vi "Pressure_statistic with temperature.vi"() -> ()   [LabVIEW 2014]
uses:
  <vilib>/Utility/error.llb/DialogType.ctl
  <instrlib>/Fluke 884X Series/Public/Data/Read (Single Point).vi
  Instance          11 26Saved   Pressure_statistic .vi
  Instance           1 26Saved   Pressure_statistic .vi
  Instance           7 26Saved   Pressure_statistic .vi
  Instance           6 26Saved   Pressure_statistic .vi
  Instance          18 26Saved   Pressure_statistic .vi
  Instance           2 26Saved   Pressure_statistic .vi
  Instance           5 26Saved   Pressure_statistic .vi
  <vilib>/Utility/file.llb/Write To Spreadsheet File (DBL).vi
  Instance           4 26Saved   Pressure_statistic .vi
  Instance           9 26Saved   Pressure_statistic .vi
  Instance           8 26Saved   Pressure_statistic .vi
  Instance          17 26Saved   Pressure_statistic .vi
  Instance          16 26Saved   Pressure_statistic .vi
  <instrlib>/Fluke 884X Series/Fluke 884X Series.lvlib
panel:
  out "Temperature from Fluke884X":dbl(graph)
  out "Temperature,V":dbl
  in  "VISA resource name":refnum<visa-resource-name>
  in  "Wire Mode (1: 4-Wire)":i16(ring)=1 items=["2-Wire", "4-Wire"]
  in  "Unit (0: Celsius)":u16(ring) items=["C", "F", "K"]
  in  "RTD Type (0: PT100_385)":u16(ring) items=["PT100_385", "PT100_392", "Custom"]
  in  "R0 (100 ohms)":i32=100
  in  "Serial Configuration":T1={"Baud Rate"=9600, "Parity"=0, "Data Bits"=8, "Stop Bits"=10, "Flow Control"=0} {"Flow Control" items=["None", "XON/XOFF", "RTS/CTS", "XON/XOFF & RTS/CTS", "DTR/DSR", "XON/XOFF & DTR/DSR"]; "Stop Bits" items=["1.0"=10, "1.5"=15, "2.0"=20]; "Data Bits" items=["7"=7, "8"=8]; "Parity" items=["None", "Odd", "Even", "Mark", "Space"]; "Baud Rate" items=["300"=300, "600"=600, "1200"=1200, "2400"=2400, "4800"=4800, "9600"=9600, "19200"=19200]}
  in  "Alpha (385)":dbl=385.0 min=374.0 max=393.0 format="%#.6p"
  in  "Filter 2":bool
  in  "Case Constant\n(See Context Help)":bool=TRUE
  in  "Write":bool
  out "T,C":dbl
  out "T,K":dbl
  in  "T, mkV":dbl
  out "P, V":dbl[](array[numeric])
  in  "Tkomn, C":dbl
  out "Waveform Graph 2":dynamicdata(graph)
  out "Waveform Graph":dynamicdata(graph)
  in  "Fourier transform":bool
  out "Pressure Frequency":dbl
  out "Pressure Amplitude":dbl
  in  "Filter":bool
  in  "Fourier transform":bool
  out "Responce Frequency":dbl
  out "Responce Amplitude":dbl
  in  "Write to file":bool
  in  "stop":bool
  # "Responce"
  # "Pressure"
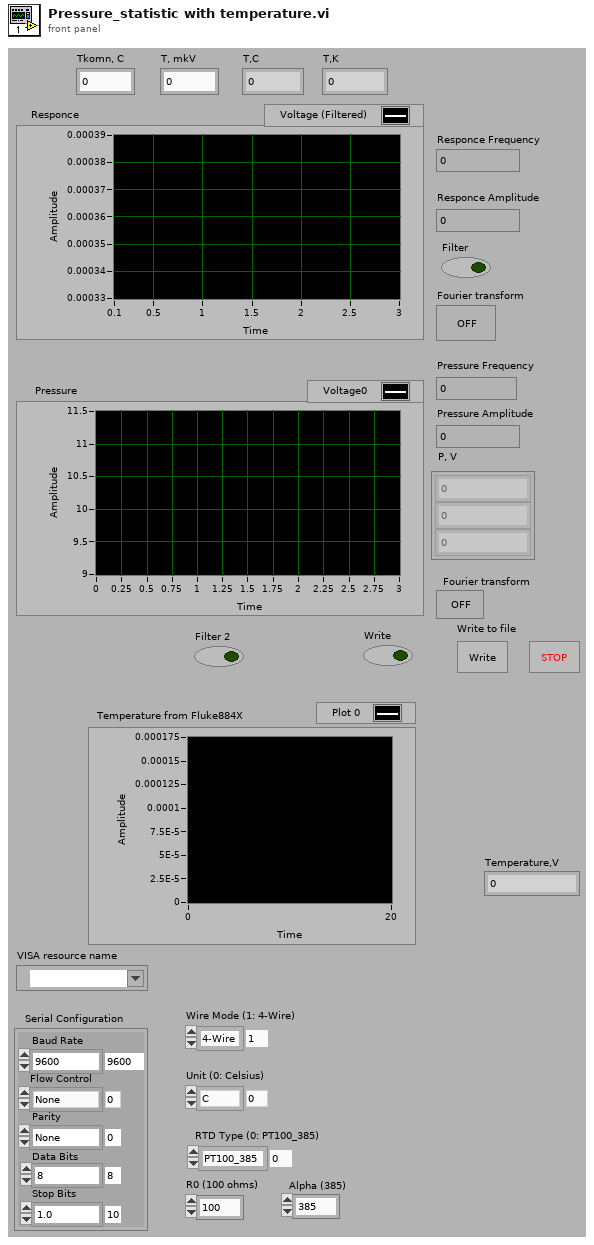
[diagram p1: front panel]
types:
  T1 = cluster{"Baud Rate":u32, "Parity":u16, "Data Bits":u16, "Stop Bits":u16, "Flow Control":u16}
  T2 = typedef "DialogType.ctl" = u16
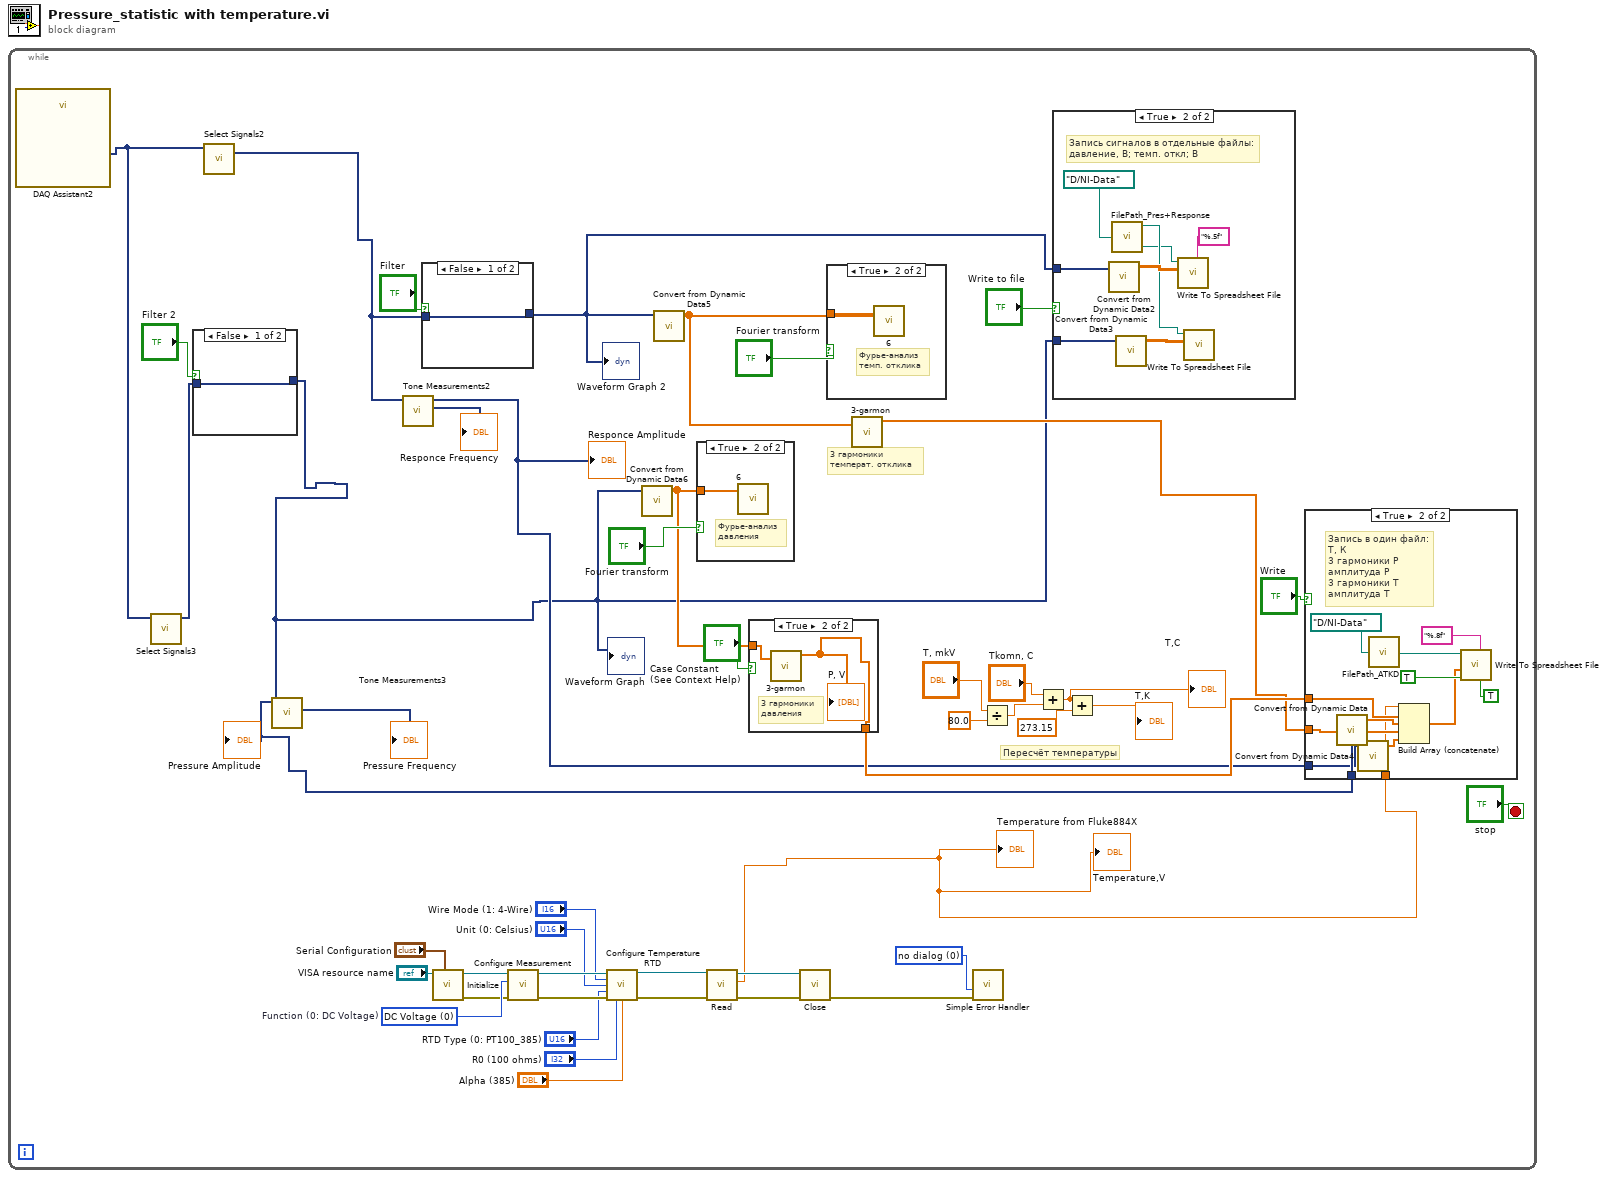
[diagram p0: block diagram]
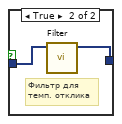
[diagram p2: hidden frame]
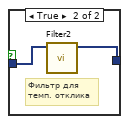
[diagram p6: hidden frame]
diagram:
  n1 = while {
    stop <- "stop" stop-if-true
    w19 = u16 0 items=["DC Voltage", "AC Voltage", "2 - Wire Resistance", "4 - Wire Resistance", "DC Current", "AC Current", "Frequency", "Period", "Continuity", "Diode Checking", "Temperature", "Capacitance"]  # Function (0: DC Voltage)
    w8 = T2 0 items=["no dialog", "OK message", "continue or stop message", "OK message + warnings", "continue/stop + warnings"] ("type of dialog (OK msg:1)")
    # "Пересчёт температуры"
    # "3 гармоники\nтемперат. отклика"
    n2 = call "DAQ Assistant2"() -> ("data"=w38:dynamicdata)  [unwired: 2 in, 9 out]
    n3 = call "Select Signals3"("Signals"=w38) -> ("Signal Out"=w23:dynamicdata)  [unwired: 1 in, 9 out]
    n4 = case shown="False" "Filter 2" {
      tunnel: w23 -> [w48 w50]
      tunnel: [w48 w49] -> w21
      frame False {
      }
      frame True {
        # "Фильтр для\nтемп. отклика"
        n5 = call "Filter"("Signal"=w50) -> ("Filtered Signal"=w49:dynamicdata)  [unwired: 2 in, 8 out]
      }
    }
    "Waveform Graph" <- w21
    n6 = call "Select Signals2"("Signals"=w38) -> ("Signal Out"=w42:dynamicdata)  [unwired: 1 in, 9 out]
    n7 = call "Tone Measurements3"("Signals"=w21) -> ("Frequency"=→"Pressure Frequency":dynamicdata, "Amplitude"=w25:dynamicdata)  [unwired: 1 in, 8 out]
    "Pressure Amplitude" <- w25
    n8 = call "Tone Measurements2"("Signals"=w42) -> ("Frequency"=→"Responce Frequency":dynamicdata, "Amplitude"=w24:dynamicdata)  [unwired: 1 in, 8 out]
    "Responce Amplitude" <- w24
    n9 = case shown="False" "Filter" {
      tunnel: w42 -> [w67 w69]
      tunnel: [w67 w68] -> w39
      frame False {
      }
      frame True {
        # "Фильтр для\nтемп. отклика"
        n10 = call "Filter2"("Signal"=w69) -> ("Filtered Signal"=w68:dynamicdata)  [unwired: 2 in, 8 out]
      }
    }
    "Waveform Graph 2" <- w39
    n11 = call <instrlib>:"Initialize.vi"("Serial Configuration"="Serial Configuration", "VISA resource name"="VISA resource name") -> ("error out"=w15:errorcluster, "VISA resource name out"=w16:refnum<visa-resource-name>)  [unwired: 8 in]
    n12 = call <instrlib>:"Configure Measurement.vi"("error in (no error)"=w15, "Function (0: DC Voltage)"=w19, "VISA resource name"=w16) -> ("error out"=w18:errorcluster, "VISA resource name out"=w17:refnum<visa-resource-name>)  [unwired: 7 in]
    n13 = call <instrlib>:"Configure Temperature RTD.vi"("VISA resource name"=w17, "Wire Mode (1: 4-Wire)"="Wire Mode (1: 4-Wire)", "Unit (0: Celsius)"="Unit (0: Celsius)", "RTD Type (0: PT100_385)"="RTD Type (0: PT100_385)", "error in (no error)"=w18, "R0 (100 ohms)"="R0 (100 ohms)", "Alpha (385)"="Alpha (385)") -> ("VISA resource name out"=w4:refnum<visa-resource-name>, "error out"=w3:errorcluster)  [unwired: 7 in]
    n14 = call "Convert from Dynamic Data6"("Dynamic Data Type"=w21) -> ("Array"=w28:dbl[])  [unwired: 3 out]
    n15 = call "Convert from Dynamic Data5"("Dynamic Data Type"=w39) -> ("Array"=w37:dbl[])  [unwired: 3 out]
    n16 = case shown="True" "Fourier transform" {
      tunnel: w28 -> [_ w66]
      frame False {
      }
      frame True {
        # "Фурье-анализ\nдавления"
        n17 = call "6.vi"("X"=w66) -> ()  [unwired: 7 out]
      }
    }
    n18 = call-poly <instrlib>:"Read.vi"("error in (no error)"=w3, "VISA resource name"=w4) -> ("error out"=w5:errorcluster, "Measurement"=w1:dbl, "VISA resource name out"=w6:refnum<visa-resource-name>)  [unwired: 7 in]
    "Temperature,V" <- w1
    "Temperature from Fluke884X" <- w1
    n19 = case shown="True" "Case Constant\n(See Context Help)" {
      tunnel: w28 -> [_ w65]
      tunnel: [_ w64] -> w27
      frame False {
      }
      frame True {
        # "3 гармоники\nдавления"
        n20 = call "3-garmon.vi"("X"=w65) -> ("A"=w64:dbl[])  [unwired: 6 out]
        "P, V" <- w64
      }
    }
    n21 = call <instrlib>:"Close.vi"("error in (no error)"=w5, "VISA resource name"=w6) -> ("error out"=w7:errorcluster)  [unwired: 9 in]
    n22 = case shown="True" "Fourier transform" {
      tunnel: w37 -> [_ w70]
      frame False {
      }
      frame True {
        # "Фурье-анализ\nтемп. отклика"
        n23 = call "6.vi"("X"=w70) -> ()  [unwired: 7 out]
      }
    }
    n24 = call "3-garmon.vi"("X"=w37) -> ("A"=w26:dbl[])  [unwired: 6 out]
    n25 = call <vilib>:"Simple Error Handler.vi"("type of dialog (OK msg:1)"=w8, "error in (no error)"=w7) -> ()  [unwired: 3 in, 5 out]
    n26 = Divide(x="T, mkV", y=80.0) -> (x/y=w33:dbl)
    n27 = Add(x="Tkomn, C", y=w33) -> (x+y=w31:dbl)
    "T,C" <- w31
    n28 = case shown="True" "Write to file" {
      tunnel: w39 -> [_ w78]
      tunnel: w21 -> [_ w75]
      frame False {
      }
      frame True {
        # "Запись сигналов в отдельные файлы:\nдавление, В; темп. откл; В"
        n29 = call "Convert from Dynamic Data2"("Dynamic Data Type"=w78) -> ("Array"=w77:dbl[][])  [unwired: 3 out]
        n30 = call "FilePath_Pres+Response.vi"("base folder path"=path "D:/NI-Data") -> ("Pressure"=w73:path, "Response"=w72:path)  [unwired: 1 out]
        n31 = call "Convert from Dynamic Data3"("Dynamic Data Type"=w75) -> ("Array"=w76:dbl[][])  [unwired: 3 out]
        n32 = call-poly <vilib>:"Write To Spreadsheet File.vi"("format (%.3f)"="%.5f", "2D data"=w77, "file path (dialog if empty)"=w72) -> ()  [unwired: 3 in, 3 out]
        n33 = call-poly <vilib>:"Write To Spreadsheet File.vi"("2D data"=w76, "file path (dialog if empty)"=w73) -> ()  [unwired: 4 in, 3 out]
      }
    }
    n34 = Add(x=w31, y=273.15) -> (x+y=→"T,K":dbl)
    n35 = case shown="True" "Write" {
      tunnel: w27 -> [_ w63]
      tunnel: w26 -> [_ w56]
      tunnel: w25 -> [_ w55]
      tunnel: w24 -> [_ w53]
      tunnel: w1 -> [_ w51]
      frame False {
      }
      frame True {
        # "Запись в один файл:\nТ, К\n3 гармоники P\nамплитуда P\n3 гармоники Т\nамплитуда Т"
        n36 = call "Convert from Dynamic Data"("Dynamic Data Type"=w55) -> ("Array"=w54:dbl[])  [unwired: 3 out]
        n37 = call "Convert from Dynamic Data4"("Dynamic Data Type"=w53) -> ("Array"=w52:dbl[])  [unwired: 3 out]
        n38 = call "FilePath_ATKD.vi"("base folder path"=path "D:/NI-Data") -> ("ATKD"=w62:path)  [unwired: 3 out]
        n39 = Build Array (concatenate)(w51, w63, w54, w56, w52) -> (w58:dbl[])
        n40 = call-poly <vilib>:"Write To Spreadsheet File.vi"("transpose? (no:F)"=TRUE, "format (%.3f)"="%.8f", "append to file? (new file:F)"=TRUE, "1D data"=w58, "file path (dialog if empty)"=w62) -> ()  [unwired: 1 in, 3 out]
      }
    }
  }
